vi "Replace IO Controls.vi"(0 "vi in":refnum<vi>, 11 "error in":errorcluster) -> (4 "vi out":refnum<vi>, 15 "error out":errorcluster)   [LabVIEW 2021, in "Converter.lvlib"]
uses:
  Converter.lvlib
  <vilib>/Utility/traverseref.llb/TRef TravTarget.ctl
  <vilib>/Utility/traverseref.llb/VI Scripting - Traverse.lvlib
  Converter Reusables/Converter Reusables.lvlib
  Path Functions/Path Functions.lvlib
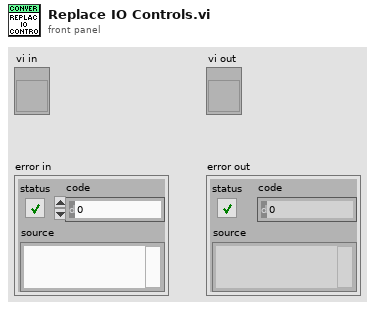
[diagram p1: front panel]
types:
  T1 = typedef "TRef TravTarget.ctl" = enum16{"FP", "BD", "Other"}
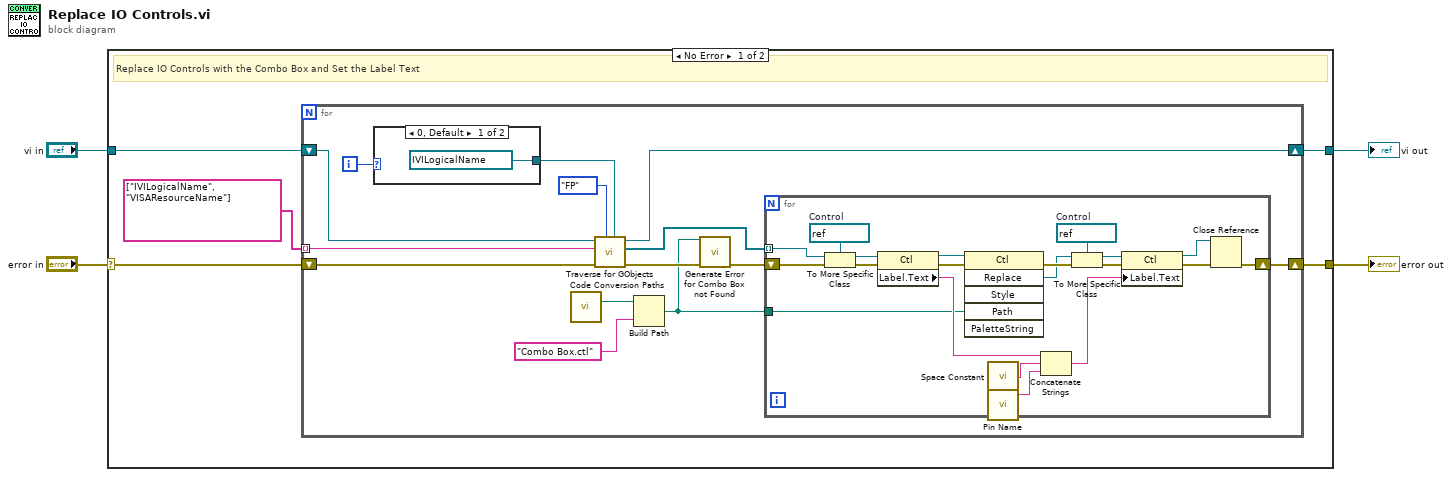
[diagram p0: block diagram]
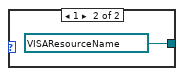
[diagram p2: hidden frame]
diagram:
  n1 = case shown="No Error" "error in" {
    selector: "error in" -> [w8 w46]
    tunnel: [w6 w46] -> w1
    tunnel: [w9 w47] -> w2
    tunnel: "vi in" -> [w7 w47]
    frame No Error {
      # "Replace IO Controls with the Combo Box and Set the Label Text"
      n2 = for {
        tunnel: string[] ["IVILogicalName", "VISAResourceName"] ("Class Name") -> [w13] mode=indexing
        shift-right: [w15] -> w6
        shift-left: w8 -> [w21]
        shift-right: [w22] -> w9
        shift-left: w7 -> [w20]
        i -> [w12]
        n3 = case shown="0, Default" w12 {
          tunnel: [refnum<vi> refnum ("Other Refnum") refnum<vi> refnum ("Other Refnum")] -> w14
          frame 0, Default {
          }
          frame 1 {
          }
        }
        n4 = call "Code Conversion Paths.vi"() -> ("io controls"=w19:path)  [unwired: 7 in, 8 out]
        n5 = call <vilib>:"Traverse for GObjects.vi"("Other Refnum"=w14, "Traverse Target"=TRef_TravTarget."FP", "error in (no error)"=w21, "Class Name"=w13, "VI Refnum"=w20) -> ("error out"=w18:errorcluster, "References"=w16:refnum<vi>[], "dup VI Refnum"=w22:refnum<vi>)  [unwired: 3 in, 1 out]
        n6 = Build Path(base path=w19, name or relative path="Combo Box.ctl" ("string")) -> (appended path=w10:path)
        n7 = call "Generate Error for Combo Box not Found.vi"("template combox path"=w10, "error in"=w18) -> ("error out"=w17:errorcluster)  [unwired: 13 in]
        n8 = for {
          tunnel: w16 -> [w43] mode=indexing
          tunnel: w10 -> [w27]
          shift-right: [w31] -> w15
          shift-left: w17 -> [w42]
          w24 = refnum<vi> refnum  # Control
          w25 = refnum<vi> refnum  # Control
          n9 = To More Specific Class(target class=w25, reference=w43, error in=w42) -> (specific class reference=w41:refnum<vi>, error out=w39:errorcluster)
          n10 = property class="Ctl"(reference=w41, error in=w39) -> (reference out=w40:refnum<vi>, error out=w38:errorcluster, "Label.Text"=w30:string)
          n11 = invoke class="Ctl" method="Replace"(reference=w40, error in=w38, "Path"=w27) -> (error out=w37:errorcluster, "Replace"=w36:refnum<vi>)  [unwired: 3 in, 4 out]
          n12 = call <vilib>:"Space Constant.vi"() -> ("String"=w29:string)
          n13 = call "Pin Name.vi"() -> ("pin name"=w28:string)  [unwired: 5 in]
          n14 = Concatenate Strings(w30, w29, w28) -> (w33:string)
          n15 = To More Specific Class(target class=w24, reference=w36, error in=w37) -> (specific class reference=w35:refnum<vi>, error out=w34:errorcluster)
          n16 = property class="Ctl"(reference=w35, error in=w34, "Label.Text"=w33) -> (reference out=w26:refnum<vi>, error out=w32:errorcluster)
          n17 = Close Reference(reference=w26, error in (no error)=w32) -> (error out=w31:errorcluster)
        }
      }
    }
    frame Error {
    }
  }
  "error out" <- w1
  "vi out" <- w2
